vi "Convert CAN Data (U8) to U32.vi"(7 "Data":u8[](array[numeric])=[1, 2, 3, 4, 5, 6, 7, 8, 9, 10, 11, 0]) -> (8 "Array":u32[](array[numeric]) format="%.0x")   [LabVIEW 2013, in "J1939.lvlib"]
uses:
  J1939.lvlib
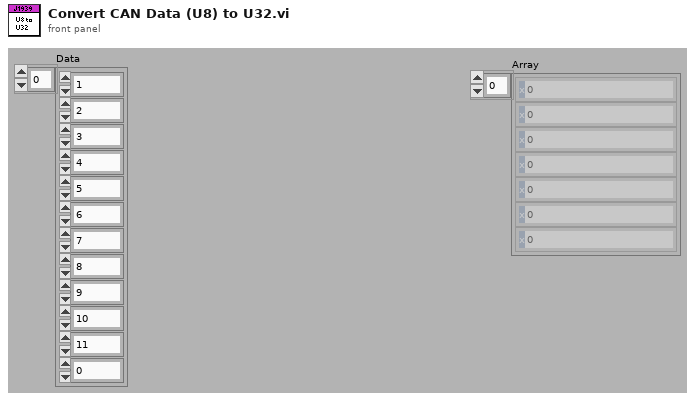
[diagram p1: front panel]
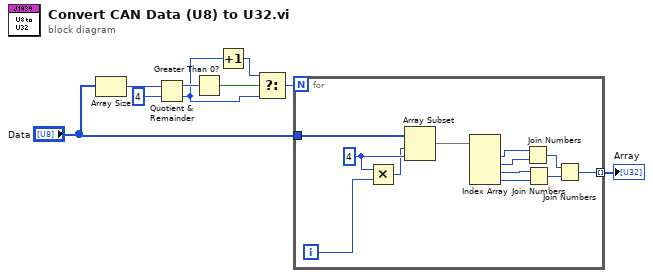
[diagram p0: block diagram]
diagram:
  n1 = Array Size(array="Data") -> (size(s)=w8:i32)
  n2 = Quotient & Remainder(x=w8, y=4) -> (x-y*floor(x/y)=w6:i32, floor(x/y)=w4:i32)
  n3 = Greater Than 0?(x=w6) -> (x > 0?=w5:bool)
  n4 = Increment(x=w4) -> (x+1=w3:i32)
  n5 = Select(t=w3, s=w5, f=w4) -> (s? t:f=w2:i32)
  n6 = for {
    N: w2 -> [_]
    tunnel: "Data" -> [w21]
    tunnel: [w13] -> w1 mode=indexing
    i -> [w12]
    w11 = 4 ("length")
    n7 = Multiply(x=w11, y=w12) -> (x*y=w10:i32)
    n8 = Array Subset(array=w21, index=w10, length=w11) -> (w20:u8[])
    n9 = Index Array(array=w20) -> (element #1=w16:u8, element #2=w17:u8, element #3=w18:u8, element #4=w19:u8)  [unwired: 4 in]
    n10 = Join Numbers(hi=w16, lo=w17) -> ((hi.lo)=w15:u16)
    n11 = Join Numbers(hi=w18, lo=w19) -> ((hi.lo)=w14:u16)
    n12 = Join Numbers(hi=w15, lo=w14) -> ((hi.lo)=w13:u32)
  }
  "Array" <- w1
